vi "AuMT8852B AFH Read FER.vi"(8 "error in (no error)":errorcluster, 11 "VISA session":refnum<visa-resource-name>) -> (0 "error out":errorcluster, 2 "error code":i32, 3 "VISA session out":refnum<visa-resource-name>, 4 "Frame Error Rate Out":dbl)   [LabVIEW 2017]
doc: "Anritsu MT8852B Bluetooth Tester\n\nReads the EUT Frame Error Rate.\nNOTE: Must follow the selection of the display screen.\n\nOUTPUTS\nFrame Error Rate Out - the current Frame Error Rate."
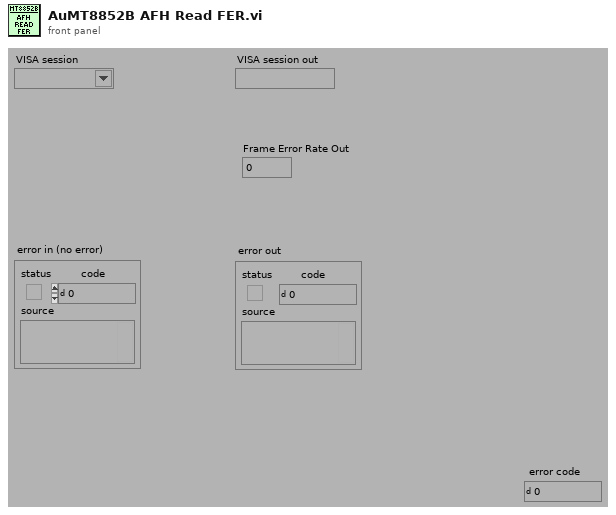
[diagram p1: front panel]
types:
  T1 = enum16{"Simulate", "Range check", "Cache", "Query instrument status"}
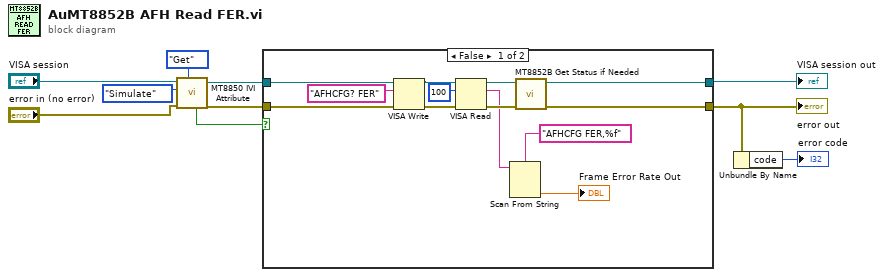
[diagram p0: block diagram]
diagram:
  n1 = call <instrlib>:"MT8850 IVI Attribute.vi"("Set/Get (Set)"=enum16{"Set", "Get"}."Get", "error in (no error)"="error in (no error)", "Flag (Simulate)"=T1."Simulate", "VISA session"="VISA session") -> ("error out"=w4:errorcluster, "VISA session out"=w5:refnum<visa-resource-name>, "Value out"=w3:bool)  [unwired: 5 in]
  n2 = case shown="False" w3 {
    tunnel: [w17 w25] -> w1
    tunnel: [w16 w24] -> w2
    tunnel: w5 -> [w22 w25]
    tunnel: w4 -> [w21 w24]
    frame False {
      n3 = VISA Write(VISA resource name=w22, write buffer="AFHCFG? FER" ("write buffer (\"\")"), error in (no error)=w21) -> (VISA resource name out=w20:refnum<visa-resource-name>, error out=w19:errorcluster)  [unwired: 1 out]
      n4 = VISA Read(VISA resource name=w20, byte count=u32 100 ("byte count (0)"), error in (no error)=w19) -> (VISA resource name out=w14:refnum<visa-resource-name>, read buffer=w13:string, error out=w15:errorcluster)  [unwired: 1 out]
      n5 = Scan From String(format string="AFHCFG FER,%f", input string=w13) -> (output 1=→"Frame Error Rate Out":dbl)  [unwired: 3 in, 3 out]
      n6 = call <instrlib>:"MT8852B Get Status if Needed.vi"("error in (no error)"=w15, "VISA session"=w14) -> ("error out"=w16:errorcluster, "VISA session out"=w17:refnum<visa-resource-name>)  [unwired: 8 in]
    }
    frame True {
    }
  }
  "error out" <- w2
  "VISA session out" <- w1
  n7 = Unbundle By Name(w2) -> ("code"=→"error code":i32)
